vi "comm status.vi"(8 "error in (no error)":errorcluster, 11 "Comm Handle":u32) -> (0 "error out":errorcluster, 1 "Error Flags":u32 format="%.0x", 2 "In Queue":u32, 3 "dup Comm Handle":u32, 4 "Status Flags":u32 format="%.0x", 6 "Out Queue":u32)   [LabVIEW 2017, in "lvserial.lvlib"]
doc: "This function retrieves information about a communications error and reports the current status of a communications device."
uses:
  lvserial.lvlib
  lvserial.dll
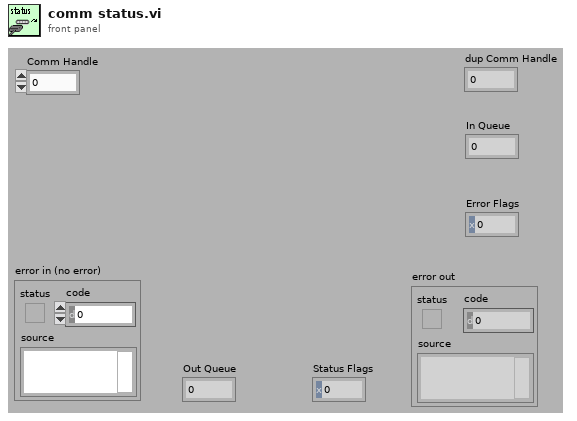
[diagram p1: front panel]
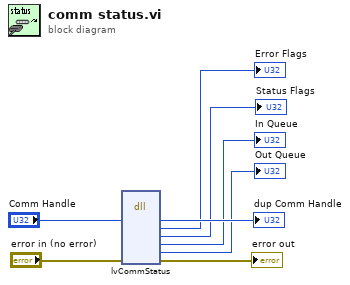
[diagram p0: block diagram]
diagram:
  n1 = dll-call lib="lvserial.dll" fn="lvCommStatus"("hComm"="Comm Handle", "error in (no error)"="error in (no error)") -> ("hComm"=→"dup Comm Handle":u32, "pulErrorFlags"=→"Error Flags":u32, "pulStatusFlags"=→"Status Flags":u32, "pulInQueue"=→"In Queue":u32, "pulOutQueue"=→"Out Queue":u32, "error in (no error)"=→"error out":errorcluster)  [unwired: 3 in, 7 out]
